vi "Send Start-Stop Message.vi"(6 "Start(T)/Stop(F)":bool, 8 "Error In":errorcluster, 9 "Version number":string, 10 "Software Name":string, 11 "Notebook Queue":refnum<queue>) -> (0 "Error Out":errorcluster)   [LabVIEW 2019, in "Notebook.lvlib"]
uses:
  Notebook.lvlib
  Notebook Action Q Element.ctl
  Notebook Action List.ctl
  Rich Text Box.lvlib
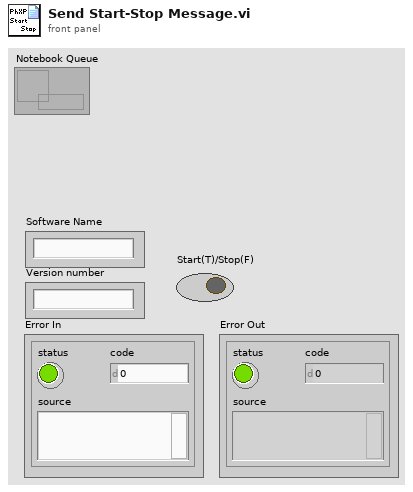
[diagram p1: front panel]
types:
  T1 = typedef "Rich Text Box.lvlib/Text Formatting.ctl" = cluster{"Font":string, "Text Color":T2, "Text Background Color":T2, "Text Style":enum16{"Regular", "Bold", "Italic", "Underline", "Strikeout"}, "Font Size (Points)":dbl, "Text Alignment":i32}
  T2 = typedef "Rich Text Box.lvlib/Text Colors.ctl" = enum16{"Unchanged", "Black", "Blue", "Gray", "Green", "Red", "White"}
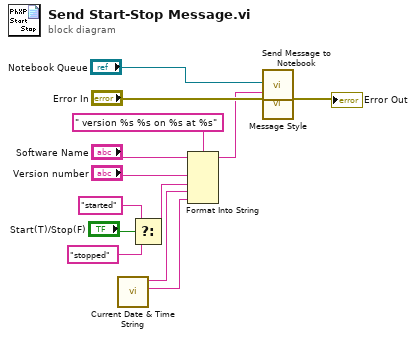
[diagram p0: block diagram]
diagram:
  n1 = call "Current Date & Time String.vi"() -> ("time string"=w2:string, "date string"=w3:string)  [unwired: 9 in, 1 out]
  n2 = Select(t="started" ("Version number"), s="Start(T)/Stop(F)", f="stopped" ("Version number")) -> (s? t:f=w6:string)
  n3 = Format Into String(format string=" version %s %s on %s at %s", initial string="Software Name", "Version number", w6, w3, w2) -> (resulting string=w5:string)  [unwired: 1 in, 1 out]
  n4 = call "Message Style.vi"() -> ("Message Formatting"=w4:T1)
  n5 = call "Send Message to Notebook.vi"("Notebook Queue"="Notebook Queue", "Message"=w5, "Error In"="Error In", "Text Formatting"=w4) -> ("Error Out"=→"Error Out":errorcluster)  [unwired: 15 in]
